vi "exercicios4_comparation.vi"() -> ()   [LabVIEW 2018]
panel:
  out "Numeric 2":dbl
  out "Resultado Final":dbl
  in  "y 2":dbl
  in  "y":dbl
  in  "x":dbl
  out "Numeric":dbl
  out "Maior que 5?":bool
  out "Palavra 1":bool
  out "Palavra 2":bool
  out "São iguais?":bool
  in  "String 2":string
  in  "String":string
  # "Exercício 1"
  # "Exercício 3"
  # "Exercício 2"
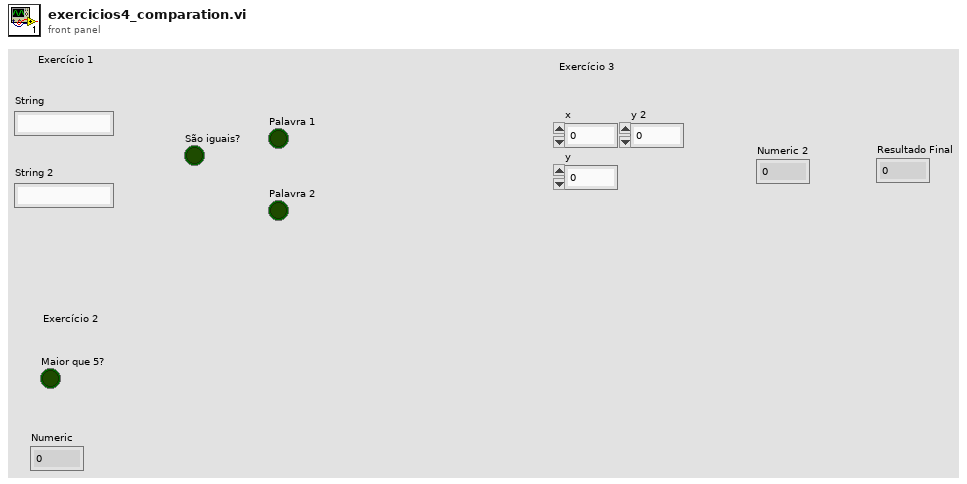
[diagram p1: front panel]
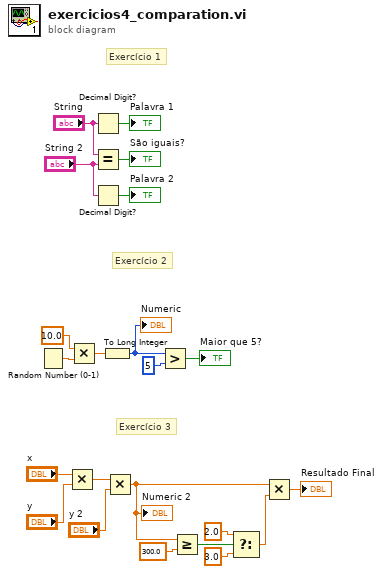
[diagram p0: block diagram]
diagram:
  # "Exercício 3"
  # "Exercício 2"
  # "Exercício 1"
  n1 = Random Number (0-1)() -> (number: 0 to 1=w17:dbl)
  n2 = Multiply(x="x", y="y") -> (x*y=w9:dbl)
  n3 = Multiply(x=10.0, y=w17) -> (x*y=w15:dbl)
  n4 = Decimal Digit?(1:"String") -> (0:→"Palavra 1":bool)
  n5 = Equal?(x="String", y="String 2") -> (x = y?=→"São iguais?":bool)
  n6 = Decimal Digit?(1:"String 2") -> (0:→"Palavra 2":bool)
  n7 = To Long Integer(number=w15) -> (32bit integer=w12:i32)
  "Numeric" <- w12
  n8 = Multiply(x=w9, y="y 2") -> (x*y=w1:dbl)
  "Numeric 2" <- w1
  n9 = Greater?(x=w12, y=5) -> (0:→"Maior que 5?":bool)
  n10 = Greater Or Equal?(x=w1, y=300.0) -> (x >= y?=w6:bool)
  n11 = Select(t=2.0, s=w6, f=3.0) -> (s? t:f=w3:dbl)
  n12 = Multiply(x=w1, y=w3) -> (x*y=→"Resultado Final":dbl)
